vi "Default Page.vi"(8 "error in":errorcluster caption="error in (no error)", 11 "Node Ptr":T1 format="%.0x") -> (0 "error out":errorcluster)   [LabVIEW 2024, in "FPGA Addon System Explorer.lvlib"]
uses:
  FPGA Addon System Explorer.lvlib
  <vilib>/NI VeriStand/Custom Device API/Custom Device Item Ref.ctl
  Parser/Custom Device Config/Custom Device Config.lvclass
  C:/dev/CD/niveristand-fpga-addon-custom-device/Source/Addon/Parser/Item/Item.lvclass
  Parser/Parser.lvlib
  <vilib>/NI VeriStand/Custom Device API/Custom Device API.lvlib
panel:
  in  "Header":cluster{"Section Name":string}={"Section Name"="FPGA Settings"}
  in  "XML Path":path
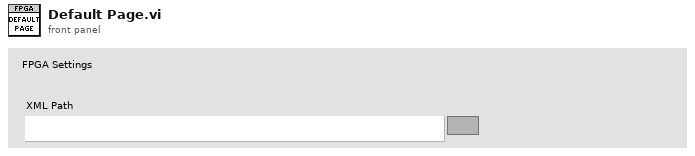
[diagram p1: front panel]
types:
  T1 = typedef "Custom Device API.lvlib/Custom Device Item Ref.ctl" = u64
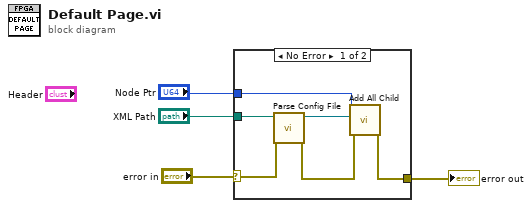
[diagram p0: block diagram]
diagram:
  n1 = case shown="No Error" "error in" {
    selector: "error in" -> [w8 w11]
    tunnel: [w9 w11] -> w4
    tunnel: "XML Path" -> [w7 _]
    tunnel: "Node Ptr" -> [w6 _]
    frame No Error {
      n2 = call "Parse Config File.vi"("error in"=w8, "XML Path"=w7) -> ("error out"=w10:errorcluster, "Custom Device Config"=w5:refnum<class "Custom Device Config.lvclass">)  [unwired: 8 in]
      n3 = call "Add All Child.vi"("error in"=w10, "Item in"=w5, "Parent Ref in"=w6) -> ("error out"=w9:errorcluster)  [unwired: 6 in, 2 out]
    }
    frame Error {
    }
  }
  "error out" <- w4
